vi "ATM_Server.vi"() -> ()   [LabVIEW 2023]
uses:
  Controller/ControllerATM.ctl
  <vilib>/Utility/file.llb/Read Delimited Spreadsheet (string).vi
  <vilib>/regexp/Match Regular Expression.xnode
panel:
  out "event error":errorcluster
  out "Output":string
  out "login error":errorcluster
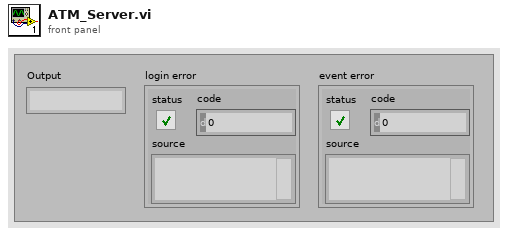
[diagram p1: front panel]
types:
  T1 = typedef "ControllerATM.ctl" = enum16{"Welcome", "Login", "Main", "Admin"}
  T2 = enum16{"open", "replace", "create", "open or create", "replace or create", "replace or create with confirmation"}
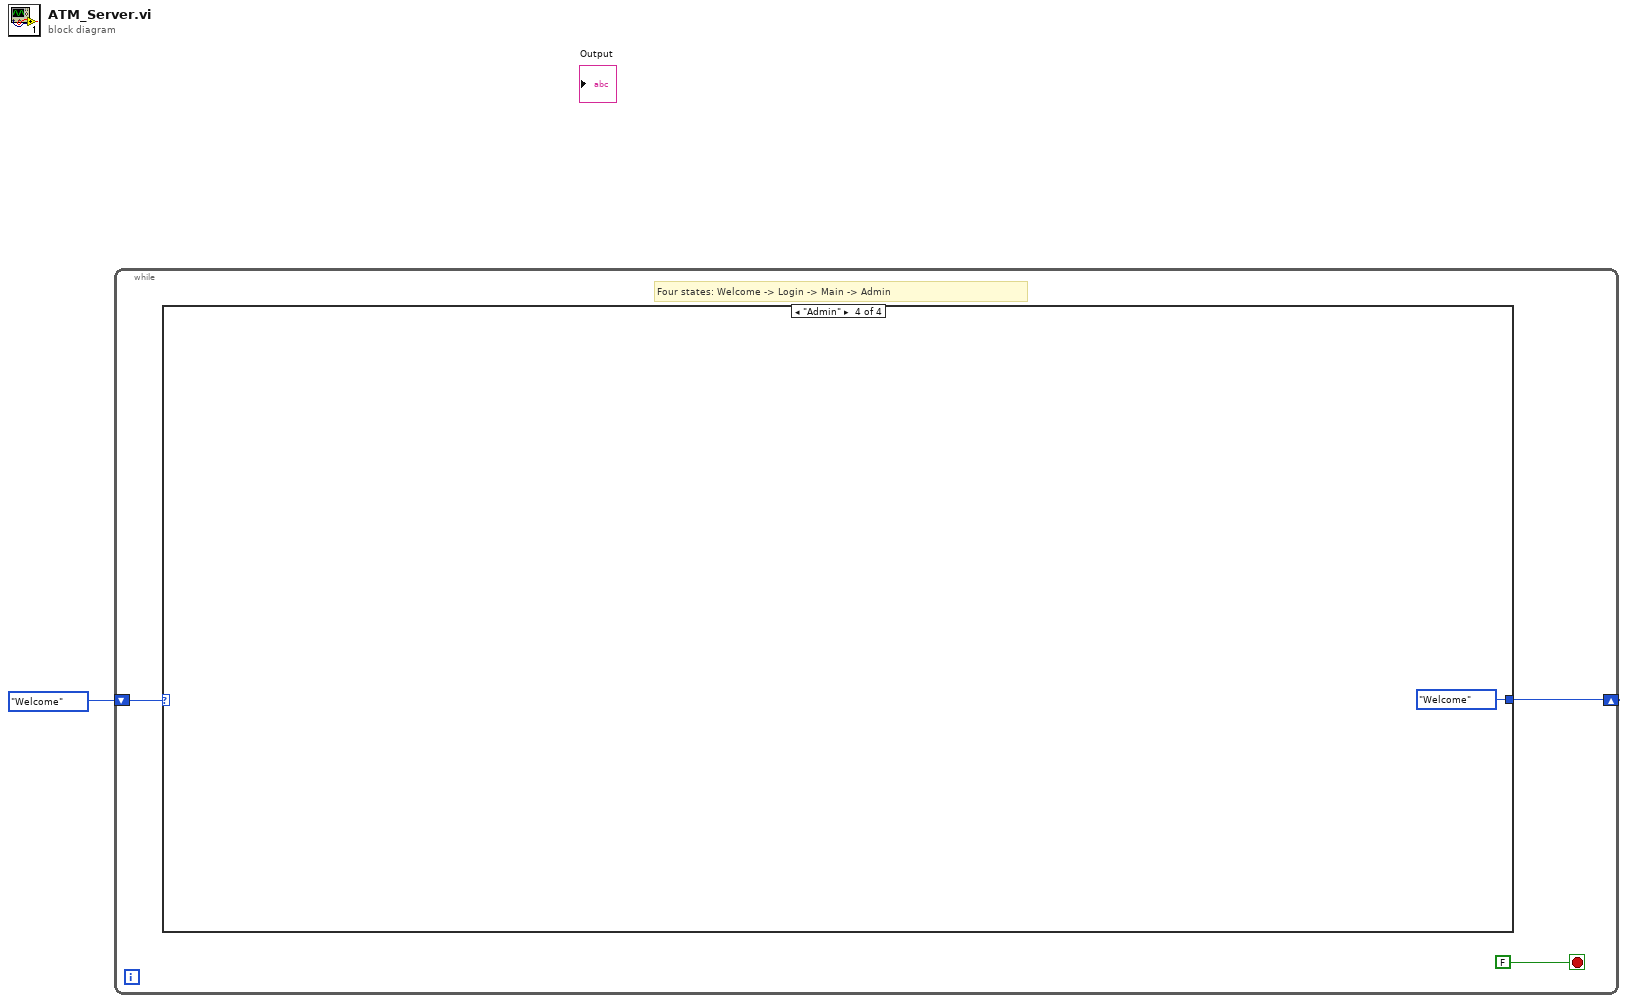
[diagram p0: block diagram]
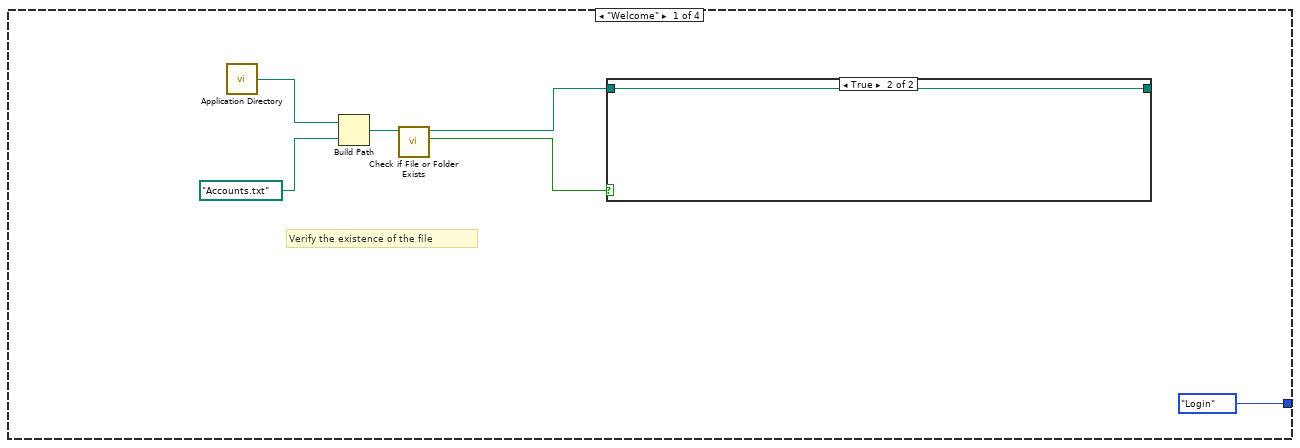
[diagram p2: hidden frame]
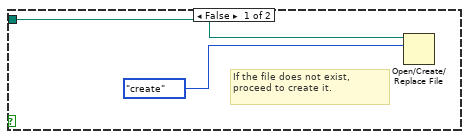
[diagram p3: hidden frame]
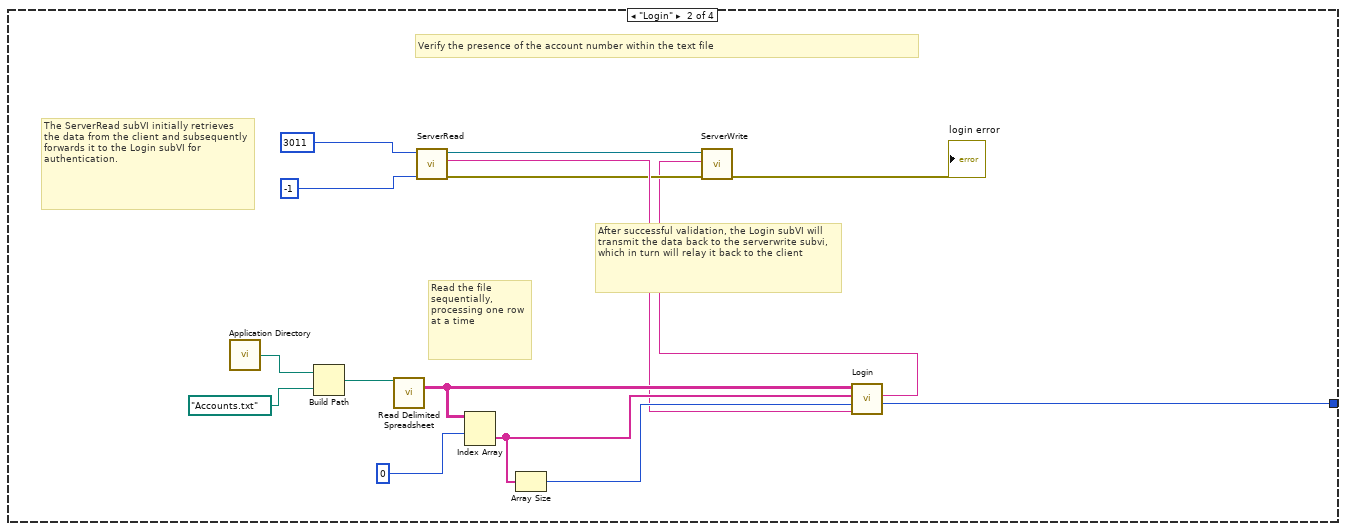
[diagram p4: hidden frame]
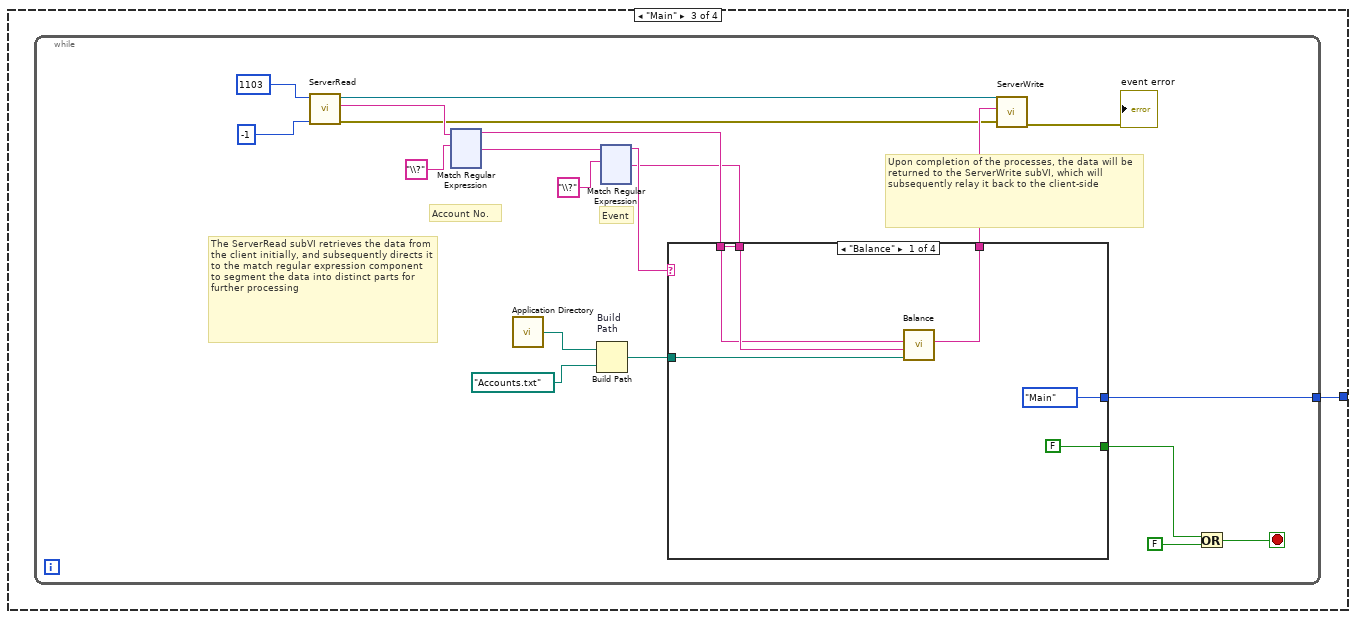
[diagram p5: hidden frame]
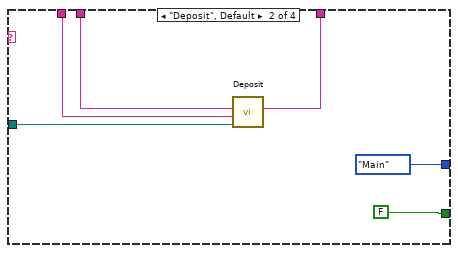
[diagram p6: hidden frame]
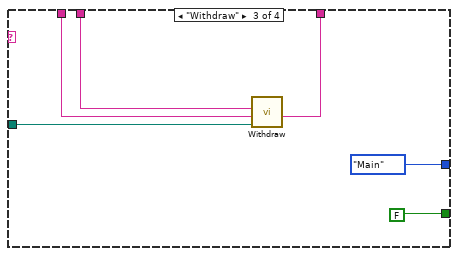
[diagram p7: hidden frame]
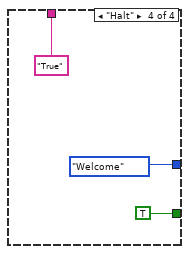
[diagram p8: hidden frame]
diagram:
  n1 = while {
    shift-right: [w3] -> _
    shift-left: ControllerATM."Welcome" -> [w2]
    stop <- FALSE stop-if-true
    # "Four states: Welcome -> Login -> Main -> Admin"
    n2 = case shown="\"Admin\"" w2 {
      tunnel: [ControllerATM."Login" w21 w29 ControllerATM."Welcome"] -> w3
      frame "Welcome" {
        # "Verify the existence of the file"
        n3 = call <vilib>:"Application Directory.vi"() -> ("Application Directory"=w9:path)
        n4 = Build Path(base path=w9, name or relative path=path "Accounts.txt") -> (appended path=w7:path)
        n5 = call <vilib>:"Check if File or Folder Exists.vi"("path"=w7) -> ("file or folder exists?"=w8:bool, "dup path"=w6:path)  [unwired: 8 in, 1 out]
        n6 = case shown="True" w8 {
          tunnel: w6 -> [w11 w13]
          tunnel: [_ w13] -> _
          frame False {
            # "If the file does not exist, \nproceed to create it."
            n7 = Open/Create/Replace File(file path (use dialog)=w11, operation (0:open)=T2."create") -> ()  [unwired: 4 in, 3 out]
          }
          frame True {
          }
        }
      }
      frame "Login" {
        # "After successful validation, the Login subVI will transmit the data back to the serverwrite subvi, which in turn will relay it back to the client"
        # "The ServerRead subVI initially retrieves the data from the client and subsequently forwards it to the Login subVI for authentication."
        # "Verify the presence of the account number within the text file"
        # "Read the file sequentially, processing one row at a time"
        n8 = call <vilib>:"Application Directory.vi"() -> ("Application Directory"=w27:path)
        n9 = Build Path(base path=w27, name or relative path=path "Accounts.txt") -> (appended path=w28:path)
        n10 = call-poly <vilib>:"Read Delimited Spreadsheet.vi"("file path (dialog if empty)"=w28) -> ("all rows"=w24:string[][])  [unwired: 9 in, 5 out]
        n11 = call "ServerRead.vi"("timeout \nms"=-1 ("timeout ms (wait forever: -1)"), "port"=u16 3011) -> ("error out"=w17:cluster{"status":bool, i32, "source":string}, "Output Data"=w18:string, "connection\n ID out"=w16:refnum<k5>)  [unwired: 7 in]
        n12 = Index Array "Index Array"(array=w24, index (col)=0 ("index (row)")) -> (element=w23:string[])  [unwired: 1 in]
        n13 = Array Size(array=w23) -> (size(s)=w22:i32)
        n14 = call "Login.vi"("data out"=w18, "Array Size"=w22, "Index Array"=w23, "2D Arrays"=w24) -> ("Enum"=w21:T1, "String"=w15:string)  [unwired: 6 in]
        n15 = call "ServerWrite.vi"("error in"=w17, "String \nInput"=w15, "connection ID"=w16) -> ("error out"=→"login error":errorcluster)  [unwired: 8 in]
      }
      frame "Main" {
        n16 = while {
          tunnel: [w41] -> w29
          stop <- w40 stop-if-true
          # "Upon completion of the processes, the data will be returned to the ServerWrite subVI, which will subsequently relay it back to the client-side"
          # "The ServerRead subVI retrieves the data from the client initially, and subsequently directs it to the match regular expression component to segment the data into distinct parts for further processing"
          # "Event"
          # "Account No."
          n17 = call "ServerRead.vi"("timeout \nms"=-1 ("timeout ms (wait forever: -1)"), "port"=u16 1103) -> ("error out"=w30:cluster{"status":bool, i32, "source":string}, "Output Data"=w34:string, "connection\n ID out"=w31:refnum<k5>)  [unwired: 7 in]
          n18 = xnode ("Match Regular \nExpression")("input string"=w34, "regular expression"="\\?") -> ("before match"=w43:string, "after match"=w48:string)  [unwired: 4 in, 3 out]
          n19 = call <vilib>:"Application Directory.vi"() -> ("Application Directory"=w46:path)
          n20 = Build Path "Build\nPath"(base path=w46, name or relative path=path "Accounts.txt") -> (appended path=w37:path)
          n21 = xnode ("Match Regular \nExpression")("input string"=w48, "regular expression"="\\?") -> ("before match"=w44:string, "after match"=w42:string)  [unwired: 4 in, 3 out]
          n22 = case shown="\"Balance\"" w44 {
            tunnel: w43 -> [w53 w58 w63 _]
            tunnel: w42 -> [w52 w59 w64 _]
            tunnel: [w54 w60 w65 "True"] -> w33
            tunnel: [ControllerATM."Main" ControllerATM."Main" ControllerATM."Main" ControllerATM."Welcome"] -> w41
            tunnel: [FALSE ("x") FALSE ("x") FALSE ("x") TRUE ("x")] -> w38
            tunnel: w37 -> [w51 w57 w62 _]
            frame "Balance" {
              n23 = call "Balance.vi"("file path"=w51, "Account No."=w53, "after match"=w52) -> ("Output"=w54:string)  [unwired: 8 in]
            }
            frame "Deposit", Default {
              n24 = call "Deposit.vi"("file path"=w57, "Account No."=w58, "Amount"=w59) -> ("Output"=w60:string)  [unwired: 8 in]
            }
            frame "Withdraw" {
              n25 = call "Withdraw.vi"("file path"=w62, "Account No."=w63, "Amount"=w64) -> ("Output"=w65:string)  [unwired: 8 in]
            }
            frame "Halt" {
            }
          }
          n26 = call "ServerWrite.vi"("error in"=w30, "String \nInput"=w33, "connection ID"=w31) -> ("error out"=→"event error":errorcluster)  [unwired: 8 in]
          n27 = Or(x=w38, y=FALSE) -> (x .or. y?=w40:bool)
        }
      }
      frame "Admin" {
      }
    }
  }
